vi "Acquire Spectrum.vi"(0 "JYCCDLib.IJYCCDReqd":refnum<k7>, 1 "Reset Plot":bool, 5 "Acq. Par.: CCD":T1={"Exposure time (ms)"=100, "Acquisition Type"=enum."Spectrum", "ADC"=0, "Gain"=10, "Shutter On/Off"=FALSE, "Number of Areas:"=1, "Area Number to Display"=1, "Show all area"=FALSE, "X Origin"=1, "X Size"=1024, "Y Origin"=1, "Y Size"=256, "Multiple Accumulations"=FALSE, "Accumulations"=1, "Number of Cleans"=1, "Shutter Mode"=3, "X Bin"=1024, "Y Bin"=256} {"Shutter Mode" items=["Open for Each Spectrum"=3, "Open for All Spectra"=1]; "Area Number to Display" min=1 max=8 step=1 format="%.0g"; "Number of Areas:" min=1 max=8 step=1; "Gain" items=["0.6x"=10, "1.0x"=11, "2.0x"=12, "4.0x"=13, "6.7x"=8, "13.3x"=2]; "ADC" items=["20 KHz"]}, 7 "CCD Dispersion":enum16{"Wavelength", "Pixel"}(ring), 9 "Calibrated Wavelength":dbl[](array[numeric]), 11 "Subtract CCD thermal background":bool, 12 "error in":errorcluster caption="Error In") -> (3 "Ref Spectrum":refnum<vi>, 4 "Max Counts":dbl, 6 "counts":dbl[](array[numeric]), 8 "Spectrum":cluster{"X":dbl[], "Y":dbl[]}[](graph), 10 "Multiple Area Spectrum":cluster{"Calibrated Wavelength":dbl[], dbl[]}[](graph), 14 "CCD Image":dbl[][](graph), 15 "Ref Multiple Area Spectrum":refnum<vi>)   [LabVIEW 2009]
panel:
  # "CCD chip area:"
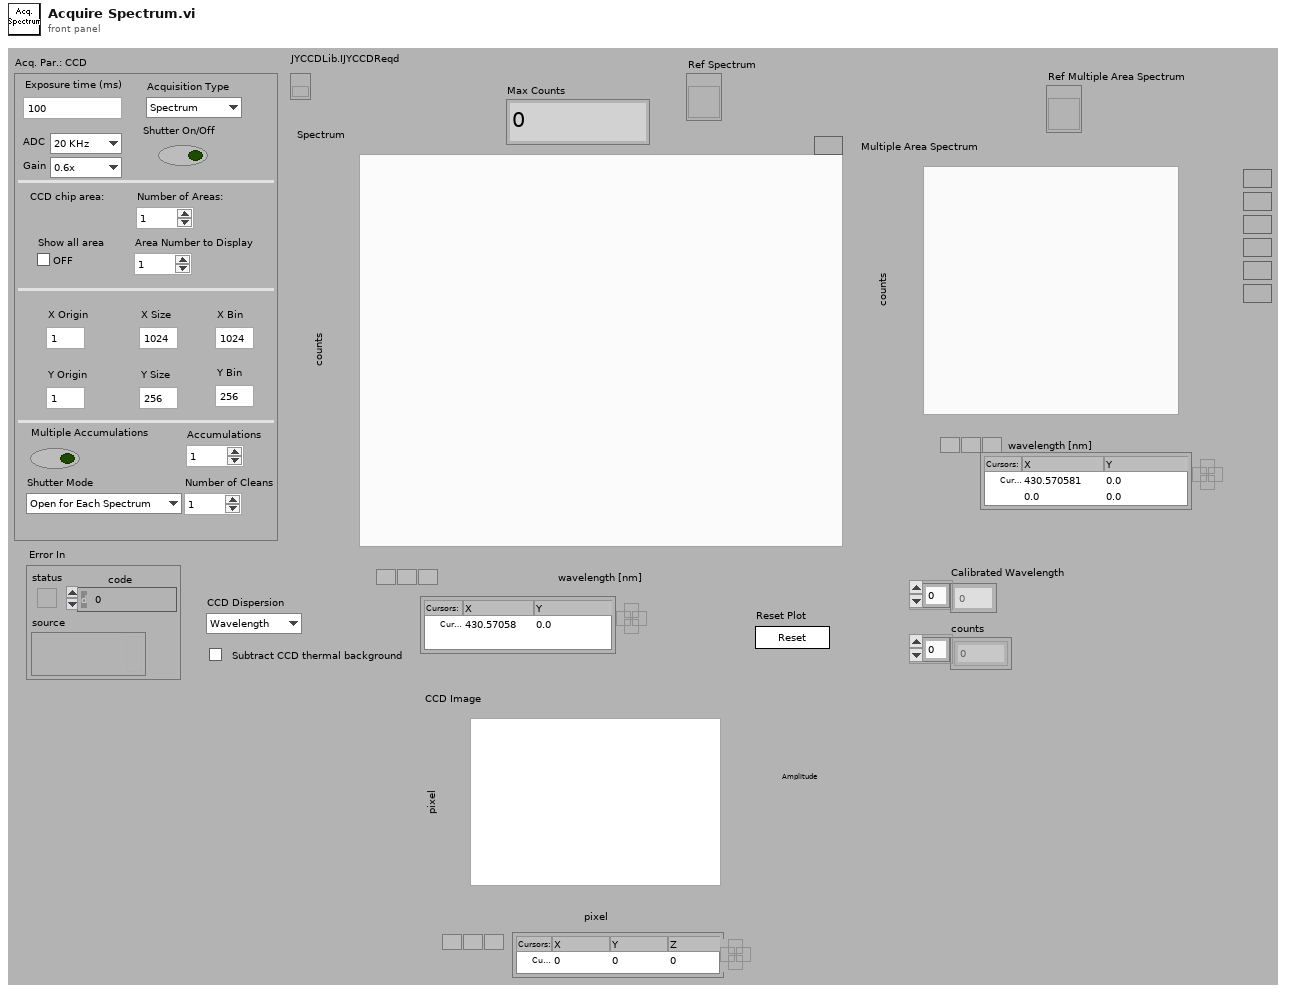
[diagram p1: front panel]
types:
  T1 = cluster{"Exposure time (ms)":i16, "Acquisition Type":enum16{"Image", "Spectrum"}, "ADC":i32, "Gain":i32, "Shutter On/Off":bool, "Number of Areas:":i32, "Area Number to Display":i32, "Show all area":bool, "X Origin":i32, "X Size":i32, "Y Origin":i32, "Y Size":i32, "Multiple Accumulations":bool, "Accumulations":i32, "Number of Cleans":i32, "Shutter Mode":i32, "X Bin":i32, "Y Bin":i32}
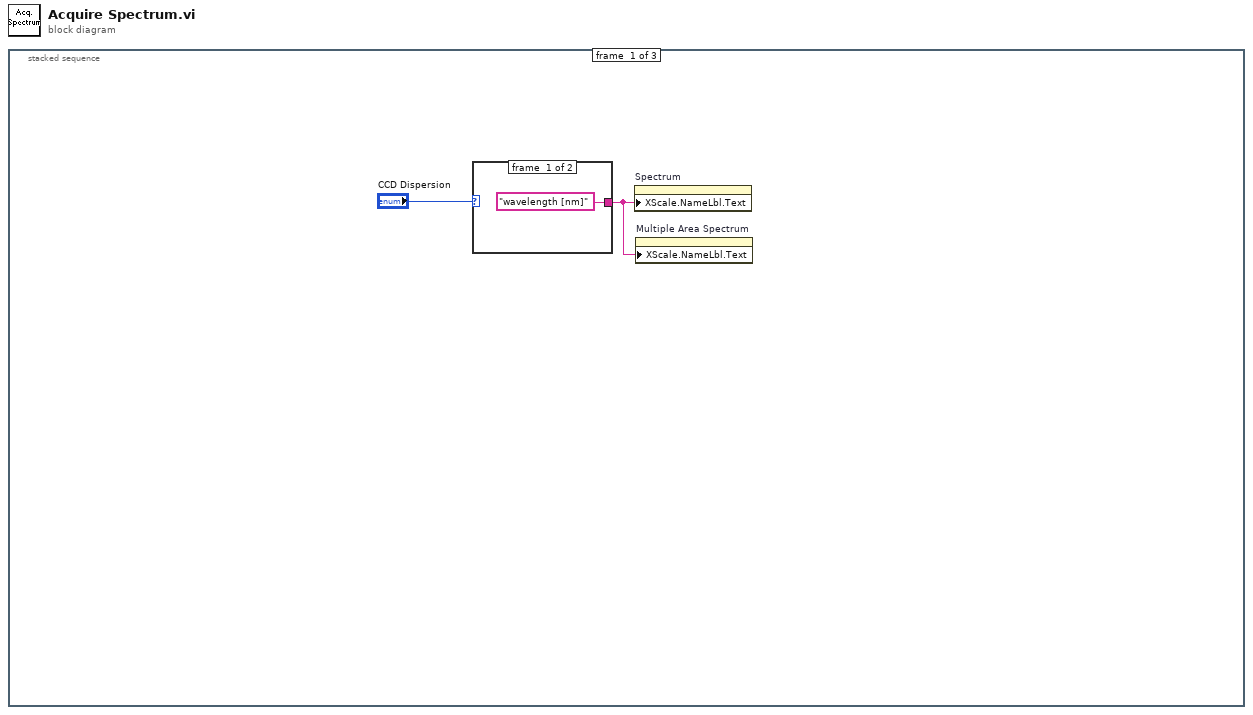
[diagram p0: block diagram]
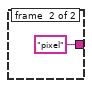
[diagram p2: hidden frame]
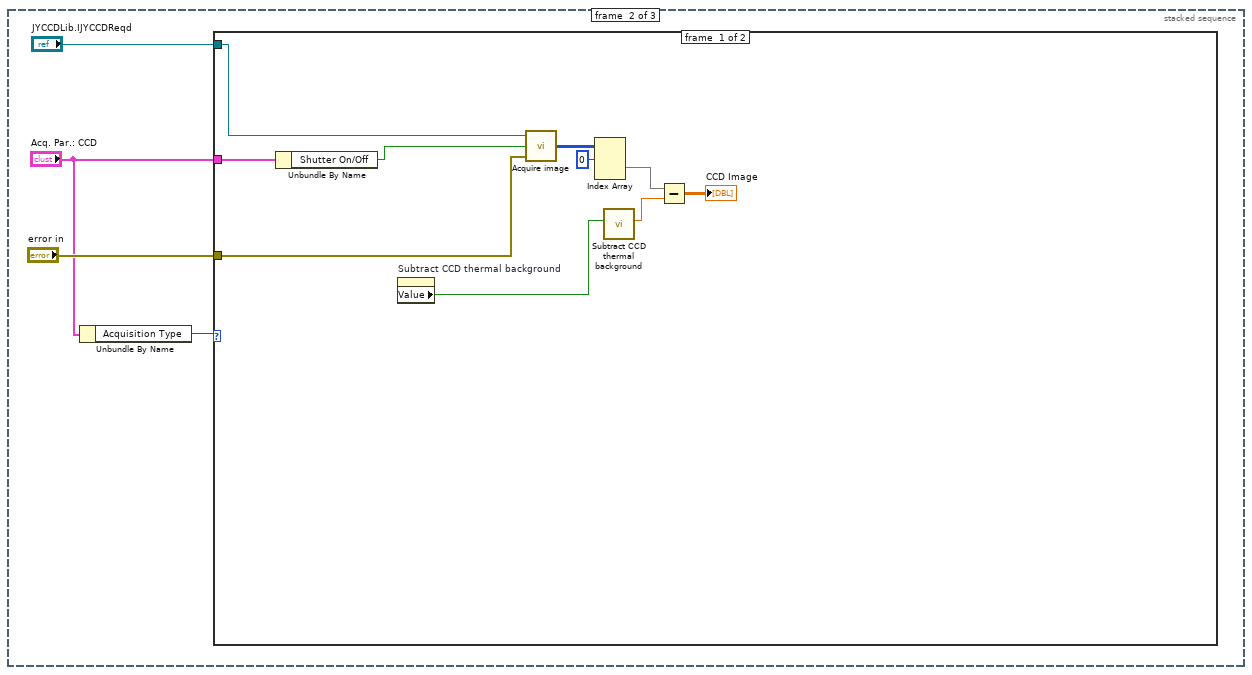
[diagram p3: hidden frame]
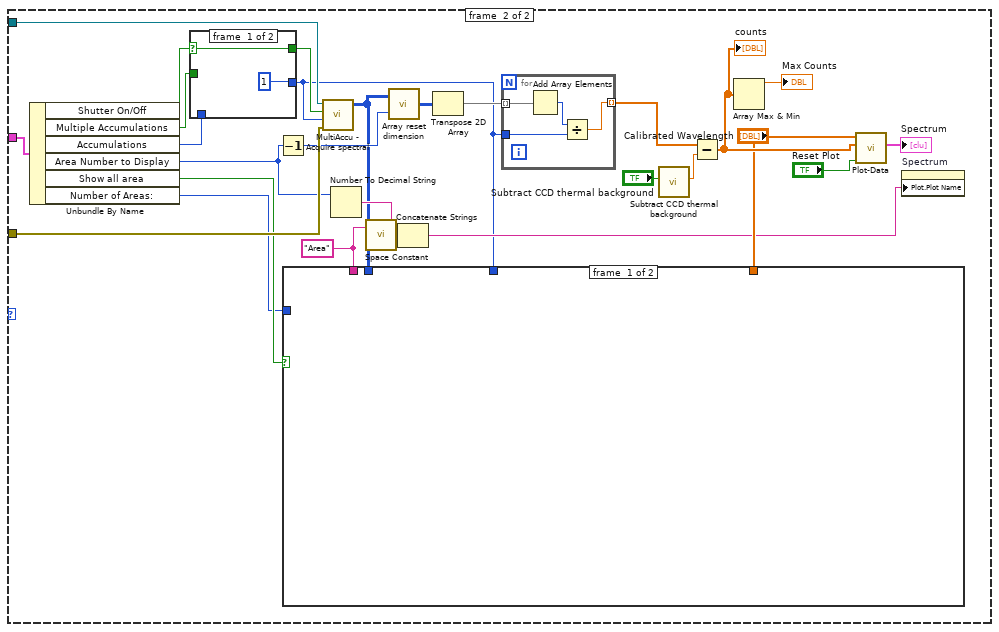
[diagram p4: hidden frame]
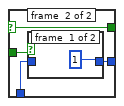
[diagram p5: hidden frame]
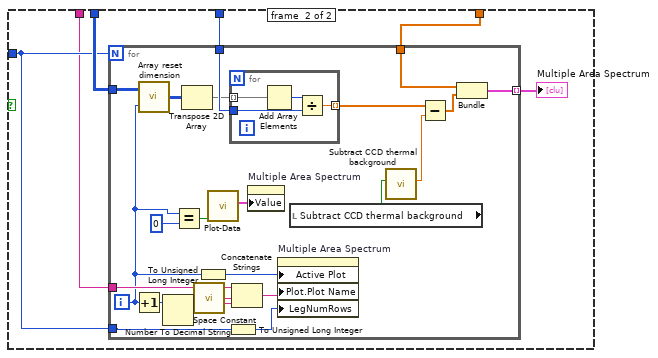
[diagram p7: hidden frame]
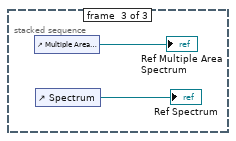
[diagram p8: hidden frame]
diagram:
  n1 = stacked-sequence {
    frame #0 {
      n2 = case shown="\"Wavelength\", Default" "CCD Dispersion" {
        tunnel: ["wavelength [nm]" "pixel"] -> w1
        frame #0 {
        }
        frame #1 {
        }
      }
      n3 = property on="Spectrum" class="XYGraph (strict)"("XScale.NameLbl.Text"=w1) -> ()  [unwired: 2 in, 2 out]
      n4 = property on="Multiple Area Spectrum" class="XYGraph (strict)"("XScale.NameLbl.Text"=w1) -> ()  [unwired: 2 in, 2 out]
    }
    frame #1 {
      n5 = Unbundle By Name("Acq. Par.: CCD") -> ("Acquisition Type"=w5:enum16{"Image", "Spectrum"})
      n6 = case shown="\"Spectrum\"" w5 {
        tunnel: "Acq. Par.: CCD" -> [w17 w45]
        tunnel: "JYCCDLib.IJYCCDReqd" -> [w18 w44]
        tunnel: "error in" -> [w15 w43]
        frame #0 {
          n7 = Unbundle By Name(w17) -> ("Shutter On/Off"=w16:bool)
          n8 = property on="Subtract CCD thermal background" class="Bool (strict)"() -> ("Value"=w9:bool)  [unwired: 2 in, 2 out]
          n9 = call "Acquire image.vi"("error in"=w15, "ShutterOpen"=w16, "JYCCDLib.IJYCCDReqd"=w18) -> ("Datas"=w14:i32[][][])  [unwired: 1 in, 1 out]
          n10 = Index Array(array=w14, index (dim 0)=0) -> (element=w11:i32[][])  [unwired: 2 in]
          n11 = call "Subtract CCD thermal background.vi"("Subtract CCD thermal background"=w9) -> ("background"=w12:dbl)  [unwired: 10 in]
          n12 = Subtract(x=w11, y=w12) -> (x-y=→"CCD Image":dbl[][])
        }
        frame #1 {
          w34 = "Area"
          n13 = Unbundle By Name(w45) -> ("Shutter On/Off"=w23:bool, "Multiple Accumulations"=w21:bool, "Accumulations"=w20:i32, "Area Number to Display"=w30:i32, "Show all area"=w39:bool, "Number of Areas:"=w29:i32)
          n14 = case shown="False" w23 {
            selector: w23 -> [w47 w51]
            tunnel: [w47 w51] -> w22
            tunnel: w21 -> [_ w50]
            tunnel: w20 -> [_ w49]
            tunnel: [1 w48] -> w19
            frame #0 {
            }
            frame #1 {
              n15 = case shown="False" w50 {
                tunnel: [1 w53] -> w48
                tunnel: w49 -> [_ w53]
                frame #0 {
                }
                frame #1 {
                }
              }
            }
          }
          n16 = Decrement(x=w30) -> (x-1=w28:i32)
          n17 = call "MultiAccu - Acquire spectral.vi"("error in"=w43, "Accumulations:"=w19, "ShutterOpen"=w22, "JYCCDLib.IJYCCDReqd"=w44) -> ("Array Out"=w27:i32[][][])  [unwired: 2 out]
          n18 = case shown="True" w39 {
            tunnel: w27 -> [_ w63]
            tunnel: w19 -> [_ w62]
            tunnel: w29 -> [_ w59]
            tunnel: "Calibrated Wavelength" -> [_ w61]
            tunnel: w34 -> [_ w58]
            frame #0 {
            }
            frame #1 {
              n19 = for {
                N: w59 -> [_]
                tunnel: w63 -> [w85]
                tunnel: w62 -> [w84]
                tunnel: w61 -> [w80]
                tunnel: [w81] -> w60 mode=indexing
                tunnel: w58 -> [w73]
                tunnel: w59 -> [w68]
                i -> [w69]
                n20 = Increment(x=w69) -> (x+1=w74:i32)
                n21 = call "Array reset dimension.vi"("Area Number"=w69, "Array In"=w85) -> ("Array Out"=w67:i32[][])
                n22 = Number To Decimal String(number=w74) -> (decimal integer string=w70:string)  [unwired: 1 in]
                n23 = Equal?(x=w69, y=0) -> (x = y?=w82:bool)
                n24 = Transpose 2D Array(2D array=w67) -> (transposed array=w66:i32[][])
                n25 = call <vilib>:"Space Constant.vi"() -> ("String"=w71:string)
                n26 = To Unsigned Long Integer(number=w69) -> (unsigned 32bit integer=w64:u32)
                n27 = call "Plot-Data.vi"("Reset Plot"=w82) -> ("Spectrum"=w75:cluster{"X":dbl[], "Y":dbl[]}[])  [unwired: 10 in]
                n28 = To Unsigned Long Integer(number=w68) -> (unsigned 32bit integer=w65:u32)
                n29 = for {
                  tunnel: w66 -> [w86] mode=indexing
                  tunnel: w84 -> [w88]
                  tunnel: [w87] -> w76 mode=indexing
                  n30 = Add Array Elements(numeric array=w86) -> (sum=w89:i32)
                  n31 = Divide(x=w89, y=w88) -> (x/y=w87:dbl)
                }
                n32 = Concatenate Strings(w73, w71, w70) -> (w72:string)
                n33 = property on="Multiple Area Spectrum" class="XYGraph (strict)"("Value"=w75) -> ()  [unwired: 2 in, 2 out]
                n34 = property on="Multiple Area Spectrum" class="XYGraph (strict)"("Active Plot"=w64, "Plot.Plot Name"=w72, "LegNumRows"=w65) -> ()  [unwired: 2 in, 2 out]
                n35 = local read "Subtract CCD thermal background"() -> (w79:bool)
                n36 = call "Subtract CCD thermal background.vi"("Subtract CCD thermal background"=w79) -> ("background"=w77:dbl)  [unwired: 10 in]
                n37 = Subtract(x=w76, y=w77) -> (x-y=w78:dbl[])
                n38 = Bundle("Calibrated Wavelength"=w80, w78) -> (w81:cluster{"Calibrated Wavelength":dbl[], dbl[]})  [unwired: 1 in]
              }
              "Multiple Area Spectrum" <- w60
            }
          }
          n39 = Number To Decimal String(number=w30) -> (decimal integer string=w32:string)  [unwired: 1 in]
          n40 = call <vilib>:"Space Constant.vi"() -> ("String"=w33:string)
          n41 = call "Array reset dimension.vi"("Area Number"=w28, "Array In"=w27) -> ("Array Out"=w26:i32[][])
          n42 = Concatenate Strings(w34, w33, w32) -> (w31:string)
          n43 = Transpose 2D Array(2D array=w26) -> (transposed array=w25:i32[][])
          n44 = for {
            tunnel: w25 -> [w57] mode=indexing
            tunnel: [w54] -> w24 mode=indexing
            tunnel: w19 -> [w55]
            n45 = Add Array Elements(numeric array=w57) -> (sum=w56:i32)
            n46 = Divide(x=w56, y=w55) -> (x/y=w54:dbl)
          }
          n47 = call "Subtract CCD thermal background.vi"("Subtract CCD thermal background"="Subtract CCD thermal background") -> ("background"=w41:dbl)  [unwired: 10 in]
          n48 = Subtract(x=w24, y=w41) -> (x-y=w37:dbl[])
          "counts" <- w37
          n49 = Array Max & Min(array=w37) -> (max value=→"Max Counts":dbl)  [unwired: 3 out]
          n50 = call "Plot-Data.vi"("Reset Plot"="Reset Plot", "Y"=w37, "X"="Calibrated Wavelength") -> ("Spectrum"=→"Spectrum":cluster{"X":dbl[], "Y":dbl[]}[])  [unwired: 8 in]
          n51 = property on="Spectrum" class="XYGraph (strict)"("Plot.Plot Name"=w31) -> ()  [unwired: 2 in, 2 out]
        }
      }
    }
    frame #2 {
      n52 = control-ref of="Multiple Area Spectrum"() -> (→"Ref Multiple Area Spectrum":refnum<vi>)
      n53 = control-ref of="Spectrum"() -> (→"Ref Spectrum":refnum<vi>)
    }
  }
